vi "VI_CmdPrompt.vi"(7 "Mode":T2, 8 "error in (no error)":errorcluster, 9 "Activate?":bool=TRUE, 10 "communication_data":T1, 11 "STR_CmdPrompt_Ref":refnum<vi>) -> (0 "error out":errorcluster)   [LabVIEW 2018]
uses:
  TypeDefs/Enum_CmdPromptActions.ctl
  OXYGEN/TypeDefs/Cluster_RawCommData.ctl
  OXYGEN.lvlib
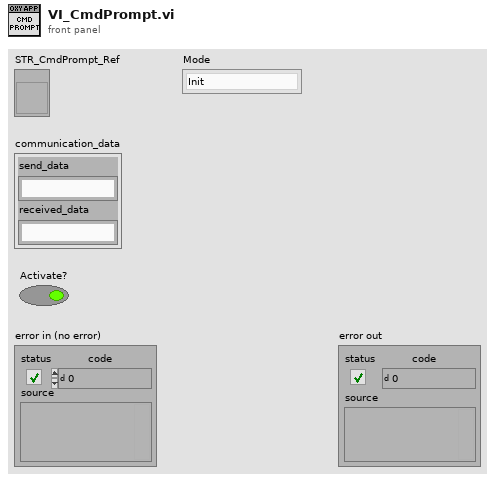
[diagram p1: front panel]
types:
  T1 = typedef "OXYGEN.lvlib/Cluster_RawCommData.ctl" = cluster{"send_data":string, "received_data":string}
  T2 = typedef "Enum_CmdPromptActions.ctl" = enum16{"Init", "Add", "EditSettings", "Close"}
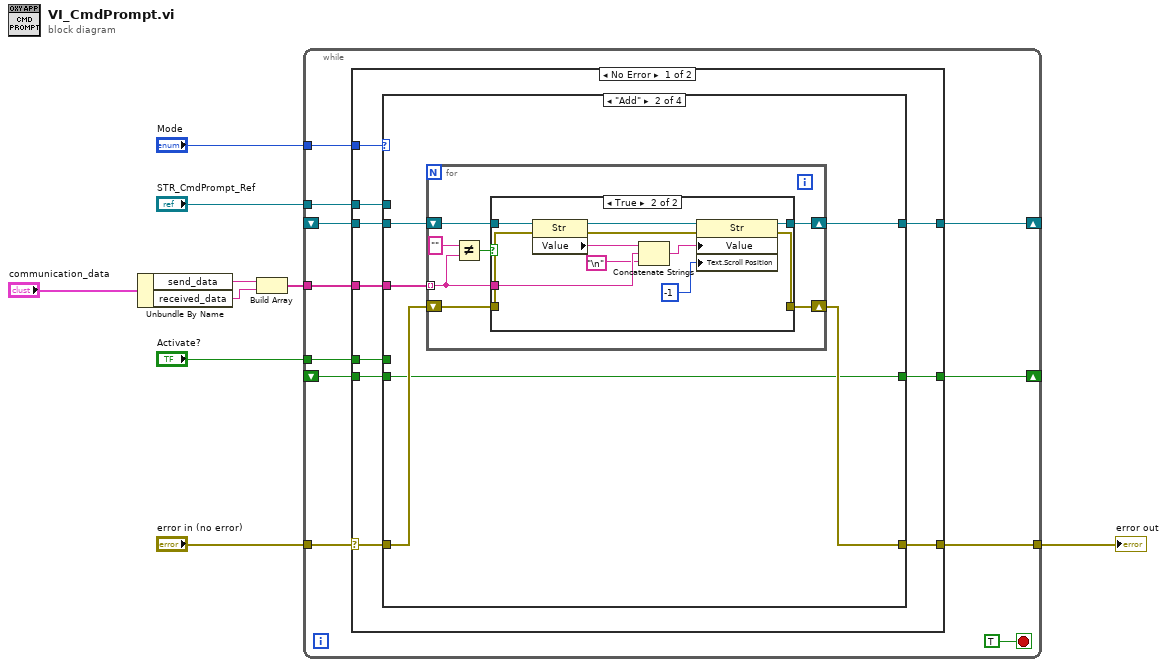
[diagram p0: block diagram]
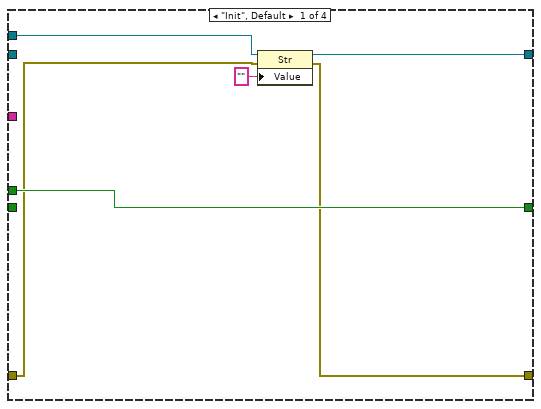
[diagram p2: hidden frame]
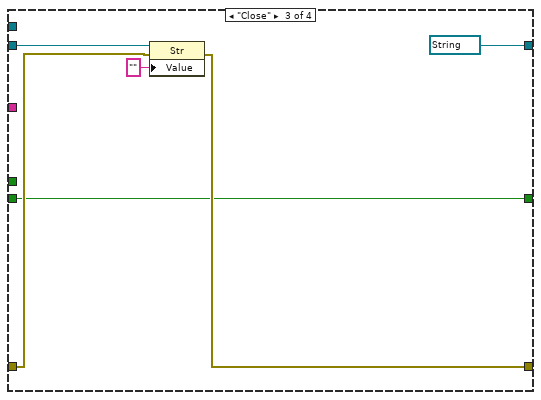
[diagram p4: hidden frame]
diagram:
  n1 = Unbundle By Name("communication_data") -> ("send_data"=w4:string, "received_data"=w3:string)
  n2 = Build Array(w4, w3) -> (w2:string[])
  n3 = while {
    tunnel: "Mode" -> [w20]
    tunnel: [w19] -> w7
    tunnel: "error in (no error)" -> [w14]
    shift-right: [w16] -> _
    shift-left: _ -> [w17]
    tunnel: w2 -> [w15]
    shift-right: [w12] -> _
    shift-left: _ -> [w13]
    tunnel: "STR_CmdPrompt_Ref" -> [w11]
    tunnel: "Activate?" -> [w10]
    stop <- TRUE stop-if-true
    n4 = case shown="No Error" w14 {
      selector: w14 -> [w25 w72]
      tunnel: w20 -> [w30 _]
      tunnel: [w29 w72] -> w19
      tunnel: w17 -> [w28 w74]
      tunnel: [w27 w74] -> w16
      tunnel: w15 -> [w26 _]
      tunnel: w13 -> [w24 w73]
      tunnel: [w23 w73] -> w12
      tunnel: w11 -> [w22 _]
      tunnel: w10 -> [w21 _]
      frame No Error {
        n5 = case shown="\"Add\"" w30 {
          tunnel: [w31 w41 w64 w69] -> w29
          tunnel: w25 -> [w32 w40 w65 w69]
          tunnel: w28 -> [_ w42 w67 w70]
          tunnel: [w34 w37 refnum<vi> refnum ("STR_CmdPrompt_Ref") w70] -> w27
          tunnel: w26 -> [_ w38 _ _]
          tunnel: w24 -> [_ w39 w63 w71]
          tunnel: [w36 w39 w63 w71] -> w23
          tunnel: w22 -> [w33 _ _ _]
          tunnel: w21 -> [w36 _ _ _]
          frame "Init", Default {
            n6 = property class="Str"(reference=w33, error in=w32, "Value"="") -> (reference out=w34:refnum<vi>, error out=w31:errorcluster)
          }
          frame "Add" {
            n7 = for {
              tunnel: w38 -> [w45] mode=indexing
              shift-right: [w47] -> w41
              shift-left: w40 -> [w46]
              shift-right: [w48] -> w37
              shift-left: w42 -> [w49]
              n8 = Not Equal?(x="", y=w45) -> (x != y?=w44:bool)
              n9 = case shown="True" w44 {
                tunnel: w49 -> [w50 w62]
                tunnel: [w50 w58] -> w48
                tunnel: [w51 w56] -> w47
                tunnel: w46 -> [w51 w55]
                tunnel: w45 -> [_ w54]
                frame False {
                }
                frame True {
                  n10 = property class="Str"(reference=w62, error in=w55) -> (reference out=w61:refnum<vi>, error out=w57:errorcluster, "Value"=w60:string)
                  n11 = Concatenate Strings(w60, w54, "\n") -> (w59:string)
                  n12 = property class="Str"(reference=w61, error in=w57, "Value"=w59, "Text.Scroll Position"=-1) -> (reference out=w58:refnum<vi>, error out=w56:errorcluster)
                }
              }
            }
          }
          frame "Close" {
            n13 = property class="Str"(reference=w67, error in=w65, "Value"="") -> (error out=w64:errorcluster)  [unwired: 1 out]
          }
          frame "EditSettings" {
          }
        }
      }
      frame Error {
      }
    }
  }
  "error out" <- w7
